vi "Configure Lock-in.vi"(8 "error in (no error)":errorcluster, 10 "Hardware Parameters":T2={"Scan Calibration [G/V]"=0.0, "Modulation Calibration [G/V]"=0.0, "Modulation Phase [deg]"=0.0, "Modulation Frequency [Hz]"=0.0, "Attenuation [dB]"=0, "Input Channel Count"=0, "Time constant"=7, "Sensitivity"=17, "Frequency Output Voltage [V]"=0.0, "Phase Output Voltage [V]"=0.0, "Lock-in Offset Compensation"=FALSE, "RF [GHz]"=0.0, "Q Start"=0.0, "Q End"=0.0, "Balance"=0.0, "Phase Error"=0.0, "AFC Error"=0.0, "AFC"=FALSE, "Magnet Rotation"=FALSE, "Balance Scaling Factor"=1.0, "Phase Error Scaling Factor"=1.0, "AFC Error Scaling Factor"=1.0, "Frequency Counter ID"="", "Sweep Waveform"=enum."Sawtooth", "Q-Factor Scale"=0.0, " Q-Data Scale"=0.0, " Q-Data Offset"=0.0, "Magnet Rotation Slope"=0.0, "Magnet Rotation Offset"=0.0, "Phase Sweep Resolution"=0.0, "Hardware Version Number"="", "Spectrometer ID Number"=0, "Spectrometer Name"="", "Lock in Saturation"=0.0, "Balance Threshold"=0.0, "Phase Error Threshold"=0.0, "AFC Error Threshold"=0.0, "Linear Actuator Length"=0.0, "Lock-in OK?"=FALSE, "Ignore Lock-in Comm. Failure"=FALSE, "Gradient Addresses"=[], "Gradient Calibrations [G/A*mm]"=[], "Gradient Power Supplies"=[], "Lock-in Address"="", "Magnet Type"=enum."RRI", "Camera Names"=[], "Sweep Limit [Gauss]"=0.0, "Modulation Limit [Gauss]"=0.0, "Balance Threshold Exceeded?"=FALSE, "Phase Threshold Exceeded?"=FALSE, "AFC Threshold Exceeded?"=FALSE, "Consecutive Re-tune attempts"=0, "Reverse Sweep Slope [sec]"=0.0, "Reverse Sweep Offset [G]"=0.0, "AFC Field Correction [V/MHz]"=0.0, "Active Gradients (X Y Z)"=[], "SpO2 Calibration [SpO2/V]"=1.0, "Heart Rate Calibration [BPM/V]"=1.0, "Thermocouple Channel"=""} {"Sensitivity" items=["", "2 nV", "5 nV", "10 nV", "20 nV", "50 nV", "100 nV", "200 nV", "500 nV", "1 uV", "2 uV", "5 uV", "10 uV", "20 uV", "50 uV", "100 uV", "200 uV", "500 uV", "1 mV", "2 mV", "5 mV", "10 mV", "20 mV", "50 mV", "100 mV", "200 mV", "500 mV", "1 V"]; "Time constant" items=["10 us", "20 us", "40 us", "80 us", "160 us", "320 us", "640 us", "5 ms", "10 ms", "20 ms", "50 ms", "100 ms", "200 ms", "500 ms", "1 s", "2 s", "5 s", "10 s", "20 s", "50 s", "100 s", "200 s", "500 s", "1 ks", "2 ks", "5 ks", "10 ks", "20 ks", "50 ks", "100 ks"]}, 11 "Acquisition Parameters":T1={"Magnet Angle [deg]"=0.0, "Magnet Angles [deg]"=[], "DeltaVpp [v]"=0.0, "SEM [v]"=0.0, "DeltaVpp Thresh [v]"=0.0, "SEM Thresh [v]"=0.0, "Adaptive Processing"=FALSE, "Acquire Q"=FALSE, "Acquire Photos"=FALSE, "Adaptive Tuning"=FALSE, "Automated Matching"=FALSE, "X-Gradient [G/mm]"=0.0, "Y-Gradient [G/mm]"=0.0, "Z-Gradient [G/mm]"=0.0, "Central Field [G]"=0.0, "Scan Width [G]"=0.0, "Mod. Amp. [G]"=0.0, "Scan Time [s]"=0.0, "Pre-Scan Delay [ms]"=0, "Measurement Timeout [s]"=0.0, "Electromagnet Main Field [G]"=0.0, "Locked Central Field [G]"=0.0, "Scans Excluded"=0, "Scans Completed"=0, "No. Scans/Set"=0, "No. Scans for SNR"=0, "Field Locked Frequency [GHz]"=0.0, "Auto Set-based Field Center"=FALSE, "Prompt for oxy acquisition updates"=FALSE, "Oxy QA Scan?"=FALSE, "Exclude Bad Data"=FALSE, "Optimizing RF Power"=FALSE, "Gradients on/off"=FALSE, "Running Script"=TRUE, "Opto-Coupler Current [A]"=0.0, "Continuous Sweeping"=FALSE, "Sweep Rise Time [sec]"=0, "Reverse Sweep Central Field [G]"=0.0, "Forward Sweep Central Field [G]"=0.0, "Sweep Calibrated"=FALSE, "Modulation Calibrated"=FALSE, "First CheckCal Scan?"=FALSE, "AFC Field Correction"=FALSE, "OxyQAInit Scan Width [G]"=0.0, "OxyQAInit Mod. Amp. [G]"=0.0, "Scans Completed/Session"=0, "Acquire SpO2"=FALSE, "Acquire Temperature"=FALSE, "Over Mod"=FALSE} {"OxyQAInit Mod. Amp. [G]" min=0.0; "OxyQAInit Scan Width [G]" min=0.0; "Mod. Amp. [G]" min=0.0; "Scan Width [G]" min=0.0; "Central Field [G]" min=0.0; "Measurement Timeout [s]" min=0.0; "Scan Time [s]" min=0.0; "Z-Gradient [G/mm]" min=0.0; "SEM Thresh [v]" min=0.0; "SEM [v]" min=0.0; "DeltaVpp [v]" min=0.0}) -> (0 "error out":errorcluster)   [LabVIEW 2016]
uses:
  Types/Hardware Parameters.ctl
  Types/Acquisition Parameters.ctl
panel:
  # "Gradients"
  # "Field"
  # "Scans and Sets"
  # "Timing"
  # "Adaptive Dosimetric \nData Processing"
  # "Bridge I/O"
  # "Magnet Rotation"
  # "Field Calibration"
  # "Lock In Amplifier"
  # "Spectrometer Information"
  # "DAQ Settings"
  # "Gradient Coils and Field"
  # "X"
  # "Y"
  # "Z"
  # "Q-Measurements"
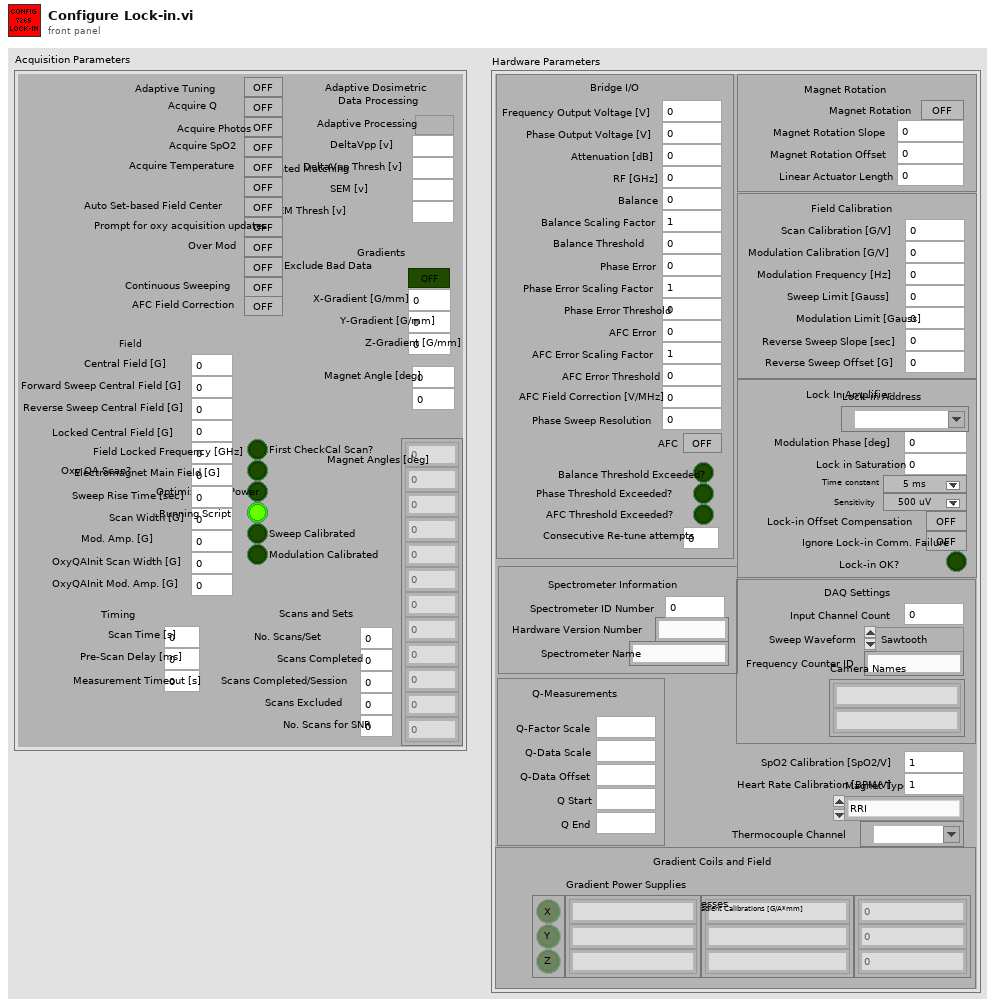
[diagram p1: front panel]
types:
  T1 = typedef "Acquisition Parameters.ctl" = cluster{"Magnet Angle [deg]":dbl, "Magnet Angles [deg]":dbl[], "DeltaVpp [v]":dbl, "SEM [v]":dbl, "DeltaVpp Thresh [v]":dbl, "SEM Thresh [v]":dbl, "Adaptive Processing":bool, "Acquire Q":bool, "Acquire Photos":bool, "Adaptive Tuning":bool, "Automated Matching":bool, "X-Gradient [G/mm]":dbl, "Y-Gradient [G/mm]":dbl, "Z-Gradient [G/mm]":dbl, "Central Field [G]":dbl, "Scan Width [G]":dbl, "Mod. Amp. [G]":dbl, "Scan Time [s]":dbl, "Pre-Scan Delay [ms]":u32, "Measurement Timeout [s]":dbl, "Electromagnet Main Field [G]":dbl, "Locked Central Field [G]":dbl, "Scans Excluded":u32, "Scans Completed":u32, "No. Scans/Set":u32, "No. Scans for SNR":u32, "Field Locked Frequency [GHz]":dbl, "Auto Set-based Field Center":bool, "Prompt for oxy acquisition updates":bool, "Oxy QA Scan?":bool, "Exclude Bad Data":bool, "Optimizing RF Power":bool, "Gradients on/off":bool, "Running Script":bool, "Opto-Coupler Current [A]":dbl, "Continuous Sweeping":bool, "Sweep Rise Time [sec]":u32, "Reverse Sweep Central Field [G]":dbl, "Forward Sweep Central Field [G]":dbl, "Sweep Calibrated":bool, "Modulation Calibrated":bool, "First CheckCal Scan?":bool, "AFC Field Correction":bool, "OxyQAInit Scan Width [G]":dbl, "OxyQAInit Mod. Amp. [G]":dbl, "Scans Completed/Session":u32, "Acquire SpO2":bool, "Acquire Temperature":bool, "Over Mod":bool}
  T2 = typedef "Hardware Parameters.ctl" = cluster{"Scan Calibration [G/V]":dbl, "Modulation Calibration [G/V]":dbl, "Modulation Phase [deg]":dbl, "Modulation Frequency [Hz]":dbl, "Attenuation [dB]":u16, "Input Channel Count":i32, "Time constant":u16, "Sensitivity":u16, "Frequency Output Voltage [V]":dbl, "Phase Output Voltage [V]":dbl, "Lock-in Offset Compensation":bool, "RF [GHz]":dbl, "Q Start":dbl, "Q End":dbl, "Balance":dbl, "Phase Error":dbl, "AFC Error":dbl, "AFC":bool, "Magnet Rotation":bool, "Balance Scaling Factor":dbl, "Phase Error Scaling Factor":dbl, "AFC Error Scaling Factor":dbl, "Frequency Counter ID":string, "Sweep Waveform":enum16{"Sine Wave", "Square Wave", "Sawtooth", "Triangle Wave"}, "Q-Factor Scale":dbl, " Q-Data Scale":dbl, " Q-Data Offset":dbl, "Magnet Rotation Slope":dbl, "Magnet Rotation Offset":dbl, "Phase Sweep Resolution":dbl, "Hardware Version Number":string, "Spectrometer ID Number":i32, "Spectrometer Name":string, "Lock in Saturation":dbl, "Balance Threshold":dbl, "Phase Error Threshold":dbl, "AFC Error Threshold":dbl, "Linear Actuator Length":dbl, "Lock-in OK?":bool, "Ignore Lock-in Comm. Failure":bool, "Gradient Addresses":string[], "Gradient Calibrations [G/A*mm]":dbl[], "Gradient Power Supplies":string[], "Lock-in Address":refnum<visa-resource-name>, "Magnet Type":enum16{"RRI", "BARDA", "Whole Body Permanent", "RRI Electromagnet"}, "Camera Names":string[], "Sweep Limit [Gauss]":dbl, "Modulation Limit [Gauss]":dbl, "Balance Threshold Exceeded?":bool, "Phase Threshold Exceeded?":bool, "AFC Threshold Exceeded?":bool, "Consecutive Re-tune attempts":i32, "Reverse Sweep Slope [sec]":dbl, "Reverse Sweep Offset [G]":dbl, "AFC Field Correction [V/MHz]":dbl, "Active Gradients (X Y Z)":bool[], "SpO2 Calibration [SpO2/V]":dbl, "Heart Rate Calibration [BPM/V]":dbl, "Thermocouple Channel":tag}
  T3 = enum16{"", "In-phase,Out-of-phase", "Magnitude, Phase"}
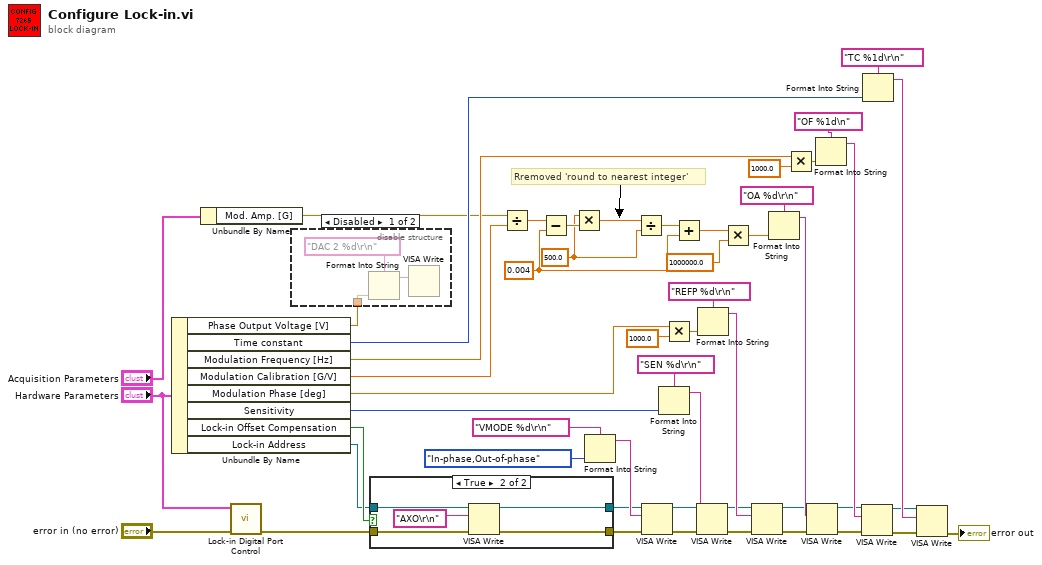
[diagram p0: block diagram]
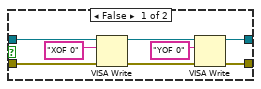
[diagram p3: hidden frame]
diagram:
  w40 = 0.004 ("y")
  w36 = 500.0 ("x")
  # "Rremoved 'round to nearest integer'"
  n1 = Unbundle By Name("Hardware Parameters") -> ("Phase Output Voltage [V]"=w2:dbl, "Time constant"=w14:u16, "Modulation Frequency [Hz]"=w13:dbl, "Modulation Calibration [G/V]"=w11:dbl, "Modulation Phase [deg]"=w10:dbl, "Sensitivity"=w9:u16, "Lock-in Offset Compensation"=w8:bool, "Lock-in Address"=w7:refnum<visa-resource-name>)
  n2 = Unbundle By Name("Acquisition Parameters") -> ("Mod. Amp. [G]"=w12:dbl)
  n3 = call "Lock-in Digital Port Control.vi"("error in (no error)"="error in (no error)", "Hardware Parameters"="Hardware Parameters") -> ("error out"=w5:errorcluster)  [unwired: 9 in]
  n4 = disable-structure shown="Disabled" {
    disable-tunnel: w2 -> [w53 _]
    frame Disabled {
      n5 = Format Into String(format string="DAC 2 %d\r\n", w53) -> (resulting string=w54:string)  [unwired: 2 in, 1 out]
      n6 = VISA Write(write buffer=w54) -> ()  [unwired: 2 in, 3 out]
    }
    frame Enabled {
    }
  }
  n7 = case shown="True" w8 {
    tunnel: [w60 w67] -> w24
    tunnel: w5 -> [w59 w65]
    tunnel: [w57 w66] -> w23
    tunnel: w7 -> [w56 w64]
    frame False {
      n8 = VISA Write(VISA resource name=w56, write buffer="XOF 0", error in (no error)=w59) -> (VISA resource name out=w63:refnum<visa-resource-name>, error out=w58:errorcluster)  [unwired: 1 out]
      n9 = VISA Write(VISA resource name=w63, write buffer="YOF 0", error in (no error)=w58) -> (VISA resource name out=w60:refnum<visa-resource-name>, error out=w57:errorcluster)  [unwired: 1 out]
    }
    frame True {
      n10 = VISA Write(VISA resource name=w64, write buffer="AXO\r\n", error in (no error)=w65) -> (VISA resource name out=w67:refnum<visa-resource-name>, error out=w66:errorcluster)  [unwired: 1 out]
    }
  }
  n11 = Divide(x=w12, y=w11) -> (x/y=w37:dbl)
  n12 = Subtract(x=w37, y=w40) -> (x-y=w38:dbl)
  n13 = Multiply(x=w36, y=w38) -> (x*y=w1:dbl)
  n14 = Format Into String(format string="VMODE %d\r\n", T3."In-phase,Out-of-phase" ("Output type")) -> (resulting string=w51:string)  [unwired: 2 in, 1 out]
  n15 = Divide(x=w1, y=w36) -> (x/y=w39:dbl)
  n16 = VISA Write(VISA resource name=w24, write buffer=w51, error in (no error)=w23) -> (VISA resource name out=w47:refnum<visa-resource-name>, error out=w22:errorcluster)  [unwired: 1 out]
  n17 = Format Into String(format string="SEN %d\r\n", w9) -> (resulting string=w49:string)  [unwired: 2 in, 1 out]
  n18 = Multiply(x=w10, y=1000.0) -> (x*y=w46:dbl)
  n19 = Add(x=w39, y=w40) -> (x+y=w41:dbl)
  n20 = VISA Write(VISA resource name=w47, write buffer=w49, error in (no error)=w22) -> (VISA resource name out=w42:refnum<visa-resource-name>, error out=w21:errorcluster)  [unwired: 1 out]
  n21 = Format Into String(format string="REFP %d\r\n", w46) -> (resulting string=w45:string)  [unwired: 2 in, 1 out]
  n22 = Multiply(x=w41, y=1000000.0 ("x")) -> (x*y=w35:dbl)
  n23 = VISA Write(VISA resource name=w42, write buffer=w45, error in (no error)=w21) -> (VISA resource name out=w31:refnum<visa-resource-name>, error out=w20:errorcluster)  [unwired: 1 out]
  n24 = Format Into String(format string="OA %d\r\n", w35) -> (resulting string=w33:string)  [unwired: 2 in, 1 out]
  n25 = Multiply(x=w13, y=1000.0) -> (x*y=w30:dbl)
  n26 = VISA Write(VISA resource name=w31, write buffer=w33, error in (no error)=w20) -> (VISA resource name out=w19:refnum<visa-resource-name>, error out=w18:errorcluster)  [unwired: 1 out]
  n27 = Format Into String(format string="OF %1d\n", w30) -> (resulting string=w29:string)  [unwired: 2 in, 1 out]
  n28 = VISA Write(VISA resource name=w19, write buffer=w29, error in (no error)=w18) -> (VISA resource name out=w17:refnum<visa-resource-name>, error out=w16:errorcluster)  [unwired: 1 out]
  n29 = Format Into String(format string="TC %1d\r\n", w14) -> (resulting string=w26:string)  [unwired: 2 in, 1 out]
  n30 = VISA Write(VISA resource name=w17, write buffer=w26, error in (no error)=w16) -> (error out=→"error out":errorcluster)  [unwired: 2 out]
